vi "RESTful HttpMethod To Text.vi"(1 "HTTP Method Type":T1) -> (0 "Boolean Text":string)   [LabVIEW 2020]
uses:
  <vilib>/AppBuilder/AB_Classes/RESTful/AB_RESTful_HTTPMethodType.ctl
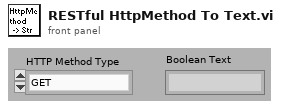
[diagram p1: front panel]
types:
  T1 = typedef "AB_RESTful_HTTPMethodType.ctl" = enum32{"GET", "POST", "PUT", "DELETE"}
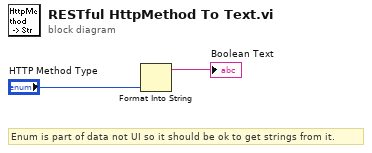
[diagram p0: block diagram]
diagram:
  # "Enum is part of data not UI so it should be ok to get strings from it."
  n1 = Format Into String("HTTP Method Type") -> (resulting string=→"Boolean Text":string)  [unwired: 3 in, 1 out]
